vi "websocket handler.vi"(9 "server information":T1, 10 "parameters":variant, 11 "upgrade data":T2) -> ()   [LabVIEW 2016, in "websocket upgrade handler.lvclass"]
uses:
  websocket upgrade handler.lvclass
  HTTP responder/http upgrade data.ctl
  lvlibtls/socket connection/lvlibretls connection.lvclass
  HTTP server/http request.ctl
  HTTP server/http method.ctl
  HTTP headers/http header data.ctl
  HTTP server/http server info.ctl
  HTTP responder/https responder.lvclass
  HTTP server/Basic HTTPS server.lvclass
  HTTP headers/http headers.lvlib
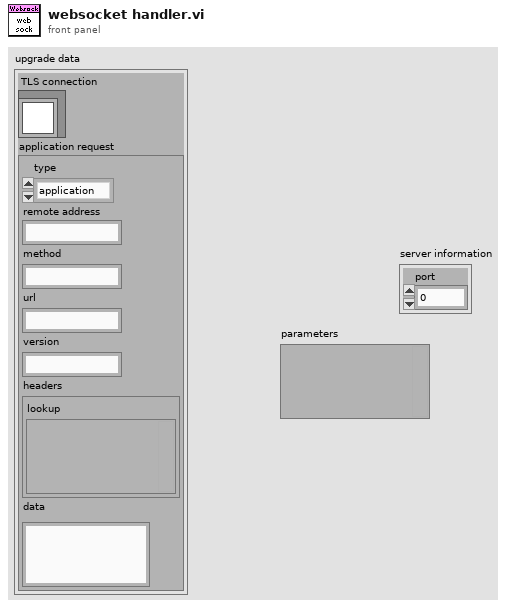
[diagram p1: front panel]
types:
  T1 = typedef "Basic HTTPS server.lvclass/http server info.ctl" = cluster{"port":u16}
  T2 = typedef "https responder.lvclass/http upgrade data.ctl" = cluster{"TLS connection":refnum<class "lvlibretls connection.lvclass">, "application request":T3}
  T3 = typedef "Basic HTTPS server.lvclass/http request.ctl" = cluster{"type":T4, "remote address":string, "method":string, "url":string, "version":string, "headers":T5, "data":string}
  T4 = typedef "Basic HTTPS server.lvclass/http method.ctl" = enum16{"application", "error", "upgrade"}
  T5 = typedef "http headers.lvlib/http header data.ctl" = cluster{"lookup":variant}
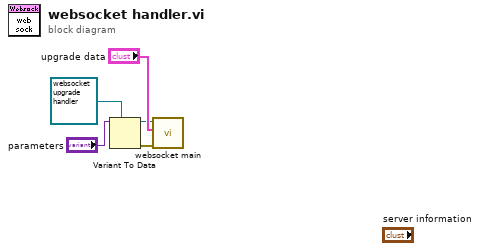
[diagram p0: block diagram]
diagram:
  n1 = Variant To Data(type=refnum<class "websocket upgrade handler.lvclass"> refnum ("websocket handler"), Variant="parameters") -> (data=w1:refnum<class "websocket upgrade handler.lvclass">, error out=w3:errorcluster)  [unwired: 1 in]
  n2 = call "websocket main.vi"("error in"=w3, "upgrade data"="upgrade data", "websocket handler in"=w1) -> ()  [unwired: 8 in, 1 out]
